vi "Motor Control Loop.vi"(8 "error in (no error)":errorcluster) -> (0 "error out":errorcluster)   [LabVIEW 2017]
uses:
  <vilib>/Simulation/Scripting/Companion Diagram/SimConfigNode/SimParams.ctl
  <vilib>/Simulation/Scripting/Companion Diagram/SimConfigNode/_simSolvers.ctl
  <vilib>/Simulation/Implementation/Shared/SIMSCR Execution Mode.ctl
  <vilib>/Platform/TimedLoop/XDataNode/timing_clust.ctl
  <vilib>/Platform/TimedLoop/XDataNode/nitl_modes.ctl
  <vilib>/Platform/TimedLoop/XDataNode/wakeup.ctl
  <vilib>/Simulation/Param Hierarchy/Typedefs/SIMPH Param Control Actions.ctl
  <vilib>/Simulation/Implementation/Shared/SIM limit type.ctl
  <vilib>/Simulation/Scripting/Editor Utilities/SIM subVI tag data.ctl
  <vilib>/Simulation/Scripting/Editor Utilities/SIM subVI execution type.ctl
  <vilib>/Simulation/Implementation/Shared/NILVSim_ParamChanged.vi
  <vilib>/Simulation/Implementation/Shared/NILVSim_FinishedLate.vi
  <vilib>/Simulation/Implementation/Shared/NILVSIM_BeginStep.vi
  <vilib>/Simulation/Utility/Implementation/SIM Halt.vi
  <vilib>/Simulation/SignalArithmetic/Implementation/NILVSim Gain.llb/SIM Gain (vector,ScalarGain).vi
  <vilib>/Simulation/ContinuousLinear/Implementation/NILVSim Integrator new.llb/SIM Integrator distributor (scalar).vi
  <vilib>/Simulation/ContinuousLinear/Implementation/NILVSim Integrator new.llb/SIM Integrator Distributor (vector).vi
  <vilib>/Simulation/Implementation/Shared/SIM Fire Discrete SubVI.vi
  <vilib>/Simulation/Nonlinear/Implementation/NILVSim Saturation.llb/SIM Saturation (scalar).vi
  <vilib>/Simulation/Nonlinear/Implementation/NILVSim Saturation.llb/SIM Saturation (vector).vi
  <vilib>/Simulation/ContinuousLinear/Implementation/NILVSim Integrator new.llb/SIM Integrator collector (scalar).vi
  <vilib>/Analysis/coordinate.llb/2D Cartesian Coordinate Rotation.vi
  <vilib>/Analysis/coordinate.llb/2D Cartesian Coordinate Rotation (Scalar).vi
  <vilib>/Simulation/ContinuousLinear/Implementation/NILVSim Integrator new.llb/SIM Integrator Collector (vector).vi
  <vilib>/Simulation/Implementation/Shared/NILVSim_Manager.vi
  <vilib>/Utility/error.llb/Clear Errors.vi
  <vilib>/Simulation/Implementation/Shared/NILVSim_FinalizeModel.vi
  <vilib>/Simulation/Implementation/Shared/SIM Fire Discrete SubVI (Core).vi
  <vilib>/robotics/Steering/Mecanum Steering Frame/NI_Robotics_Mecanum Steering Frame.lvclass
  c:/Program Files (x86)/National Instruments/LabVIEW 2017/vi.lib/robotics/Steering/Steering Frame/NI_Robotics_Steering Frame.lvclass
  <vilib>/Simulation/Implementation/Shared/SIM Unbundle Sim Info.vi
  <vilib>/Simulation/Implementation/Shared/SIMSH Read Queue.vi
  Robot Parameters/Robot Parameters.vi
  <vilib>/Simulation/Implementation/Shared/NILVSim_Initialize.vi
  <vilib>/Simulation/Utility/Implementation/NILVSim Get Time and IsAcceptedStep.vi
  Simulation/Global - Real Position.vi
  <vilib>/robotics/Steering/Steering Frame/Apply Velocity to Motors.vi
  <vilib>/robotics/Steering/Steering Frame/Apply Steering Frame Velocity to Motors.vi
  Unsaturate Commanded Motor Velocities.vi
  <vilib>/robotics/Steering/Steering Frame/Get Velocity from Motors.vi
  <vilib>/robotics/Steering/Steering Frame/Get Steering Frame Velocity from Motors.vi
  <vilib>/Simulation/Implementation/Shared/NILVSim_GetModelError.vi
  <vilib>/Simulation/Implementation/Shared/SIM Bundle Sim Info.vi
  <vilib>/Simulation/Scripting/Companion Diagram/SimConfigNode/SimDog.xnode
  PID_scalar (derivative acts only on process variable).vi
  Simulation/Mecanum Robot Body Model.vi
  Simulation/Motor Model.vi
  Simulation/PID_vector (derivative acts only on process variable).vi
  <vilib>/Platform/TimedLoop/XDataNode/XDataNode.xnode
  <vilib>/Simulation/Implementation/XNodeFramework/SimXNode/SimX.xnode
  <vilib>/robotics/Utilities/NI_Robotics Utilities.lvlib
  <vilib>/Analysis/NI_AALPro.lvlib
  <vilib>/robotics/Steering/Steering Frame/NI_Robotics_Steering Frame.lvclass
  c:/Program Files (x86)/National Instruments/LabVIEW 2017/vi.lib/robotics/Steering/Special Steering Frame/NI_Robotics_Special Steering Frame.lvclass
  <vilib>/Simulation/ContinuousLinear/Implementation/NILVSim Integrator new.llb/SIM Integrator (scalar).vi
  <vilib>/Simulation/ContinuousLinear/Implementation/NILVSim Integrator new.llb/SIM Integrator (vector).vi
  <vilib>/Platform/TimedLoop/XDataNode/XDNodeRunTimeDep.lvlib
  <vilib>/Simulation/Implementation/Shared/NI_SIM_Implementation.lvlib
panel:
  in  "stop?":bool
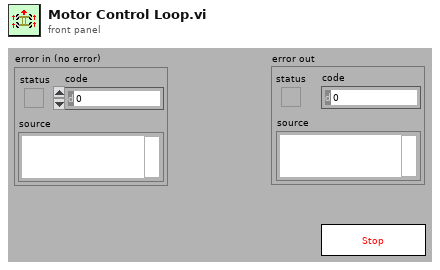
[diagram p1: front panel]
types:
  T1 = typedef "SIMSCR Execution Mode.ctl" = enum16{"Simulate to Completion", "Single Time-Step Simulation (Fixed Step Only)"}
  T2 = typedef "XDNodeRunTimeDep.lvlib/timing_clust.ctl" = cluster{"Expected End [f-1]":u64, "Actual End [f-1]":u64, "Finished Late? [f-1]":bool, "Expected End [i-1]":u64, "Actual End [i-1]":u64, "Finished Late? [i-1]":bool, "Expected Start [i]":u64, "Actual Start [i]":u64, "Expected Start [f]":u64, "Actual Start [f]":u64, "Source Name":string, "Structure Name":string, "Period":i64, "Deadline":i64, "Offset":i64, "Start":i64, "Priority":i32, "Timeout":i32, "Mode":T3, "Wakeup Reason":T4, "Error":errorcluster, "Source Type":string, "Secondary Source Type":string, "Global End Time":u64, "Global Start Time":u64, "Frame Duration":u64, "Iteration Duration":u64, "Assigned CPU":i32, "I/O Scan Engine Mode":u32}
  T3 = typedef "XDNodeRunTimeDep.lvlib/nitl_modes.ctl" = enum32{"No Change", "Process missed periods, maintain original phase", "Discard missed periods, maintain original phase", "Process missed periods, ignore original phase", "Discard missed periods, ignore original phase"}
  T4 = typedef "XDNodeRunTimeDep.lvlib/wakeup.ctl" = enum32{"Normal", "Aborted", "Asynchronous wakeup", "Timing source error", "Timed loop error", "Timeout"}
  T5 = typedef "SIMPH Param Control Actions.ctl" = enum16{"get params", "set params"}
  T6 = typedef "SIM subVI tag data.ctl" = cluster{"period":dbl, "skew":dbl, "Simulation execution type":T7}
  T7 = typedef "SIM subVI execution type.ctl" = enum16{"Function call", "Discrete", "Continuous", "Initialization only", "Final step only"}
  T8 = typedef "SIM limit type.ctl" = enum16{"upper", "lower", "both", "none"}
  T9 = cluster{"SIMSH Sim Time":dbl, "Integrator":cluster{"output":dbl}, "Gain":cluster{"output":dbl}, "Summation":cluster{"Result":dbl}, "Derivative":cluster{"output":dbl}, "Multiply":cluster{"x*y":dbl}, "Negate":cluster{"-x":dbl}, "Subtract":cluster{"x-y":dbl}, "set point":dbl, "Divide":cluster{"x/y":dbl}}
  T10 = cluster{"SIMSH Sim Time":dbl, "w":cluster{"output":dbl}, "theta":cluster{"output":dbl}, "x'":cluster{"output":dbl[]}, "x":cluster{"output":dbl[]}, "Wheel theta":cluster{"output":dbl[]}, "Robot Parameters.vi 7":cluster{"mass":dbl}, "Robot Parameters.vi 6":cluster{"inertia (Izz)":dbl}, "Robot Parameters.vi 5":cluster{"center of mass y":dbl}, "Robot Parameters.vi 4":cluster{"center of mass x":dbl}, "Robot Parameters.vi 3":cluster{"robot length":dbl}, "Robot Parameters.vi 2":cluster{"robot width":dbl}, "Robot Parameters.vi":cluster{"wheel radius":dbl}, "Divide 5":cluster{"x/y":dbl[]}, "A x B.vi 3":cluster{"A x Vector":dbl[]}, "Build Array":cluster{"appended array":dbl[]}, "Multiply 6":cluster{"x*y":dbl}, "Divide 4":cluster{"x/y":dbl}, "Add 4":cluster{"x+y":dbl}, "Index Array 4":cluster{"element":dbl}, "2D Cartesian Coordinate Rotation.vi 3":cluster{"y out":dbl, "x out":dbl}, "Multiply 5":cluster{"x*y":dbl}, "Multiply 4":cluster{"x*y":dbl}, "Add 3":cluster{"x+y":dbl}, "Add 2":cluster{"x+y":dbl}, "2D Cartesian Coordinate Rotation.vi 2":cluster{"y out":dbl, "x out":dbl}, "Replace Array Subset 2":cluster{"output array":dbl[]}, "Index Array 3":cluster{"element":dbl}, "Add":cluster{"x+y":dbl}, "Compound Arithmetic":cluster{"result":dbl}, "Multiply 3":cluster{"x*y":dbl}, "Multiply 2":cluster{"x*y":dbl}, "Multiply":cluster{"x*y":dbl}, "Index Array 2":cluster{"element":dbl}, "A x B.vi 2":cluster{"A x Vector":dbl[]}, "Divide 3":cluster{"x/y":dbl[]}, "A x B.vi":cluster{"A x Vector":dbl[]}, "Divide 2":cluster{"x/y":dbl[]}, "Replace Array Subset":cluster{"output array":dbl[]}, "Negate":cluster{"-x":dbl}, "Index Array":cluster{"element":dbl}, "2D Cartesian Coordinate Rotation.vi":cluster{"y out":dbl, "x out":dbl}, "Divide":cluster{"x/y":dbl}}
  T11 = cluster{"SIMSH Sim Time":dbl, "Gain":cluster{"output":dbl[]}, "Summation 2":cluster{"Result":dbl[]}, "Shaft Angle":cluster{"output":dbl[]}}
  T12 = cluster{"SIMSH Sim Time":dbl, "Integrator":cluster{"output":dbl[]}, "Gain":cluster{"output":dbl[]}, "Summation":cluster{"Result":dbl[]}, "Derivative":cluster{"output":dbl[]}, "Multiply":cluster{"x*y":dbl[]}, "Negate":cluster{"-x":dbl[]}, "Subtract":cluster{"x-y":dbl[]}, "set point":dbl[], "Divide":cluster{"x/y":dbl[]}}
  T13 = typedef "SimParams.ctl" = cluster{"Initial Time (s)":dbl, "Final Time (s)":dbl, "Step Size (s)":dbl, "ODE Solver":T14, "Minimum Step Size (s)":dbl, "Maximum Step Size (s)":dbl, "Relative Tolerance":dbl, "Absolute Tolerance":dbl, "Software Timing":bool, "Initial Step Size (s)":dbl, "Automatic Fixed Step Size?":bool, "Automatic Discrete Step Size?":bool, "Discrete Step Size (s)":dbl, "Calculate using Time Step":bool, "Solver Wired?":bool, "Prev.Frm.Expected End":u64, "Prev.Frm.Actual End":u64, "Prev.Frm.Finished Late?":bool, "Prev.Iter.Expected End":u64, "Prev.Iter.Actual End":u64, "Prev.Iter.Finished Late?":bool, "Expected Iteration Start":u64, "Actual Iteration Start":u64, "Expected Frame Start":u64, "Actual Frame Start":u64, "Source Name":string, "Name":string, "Period":i64, "Deadline":i64, "Offset":i64, "Start":i64, "Priority":i32, "Timeout":i32, "Processor":i32, "Mode":enum32{"No Change", "Process missed periods, maintain original phase", "Discard missed periods, maintain original phase", "Process missed periods, ignore original phase", "Discard missed periods, ignore original phase"}, "Wakeup reason":enum32{"Normal", "Aborted", "Asynchronous wakeup", "Timing source error", "Timed loop error", "Timeout"}, "Error":errorcluster, "Source Type":string, "Secondary Source Type":string, "Global End Time":u64, "Global Start Time":u64, "Full Solver Reset":bool, "Execution Mode":T1, "Nan/Inf Check":bool, "Custom Solver Library":string, "Solver Is Variable":bool, "custom solver name":string, "Signal Collection Decimation":u32}
  T14 = typedef "_simSolvers.ctl" = enum16{"Runge-Kutta 1 (Euler)", "Runge-Kutta 2", "Runge-Kutta 3", "Runge-Kutta 4", "Runge-Kutta 23 (variable)", "Runge-Kutta 45 (variable)", "BDF (variable)", "Adams-Moulton (variable)", "Rosenbrock (variable)", "Discrete States Only", "SDIRK 4 (variable)", "Radau 5 (variable)", "Radau 9 (variable)", "Radau 13 (variable)", "Radau [Variable Order] (variable)", "Gear's Method (variable)", "Linearizer", "State Query", "Trim Eval", "Custom Solver"}
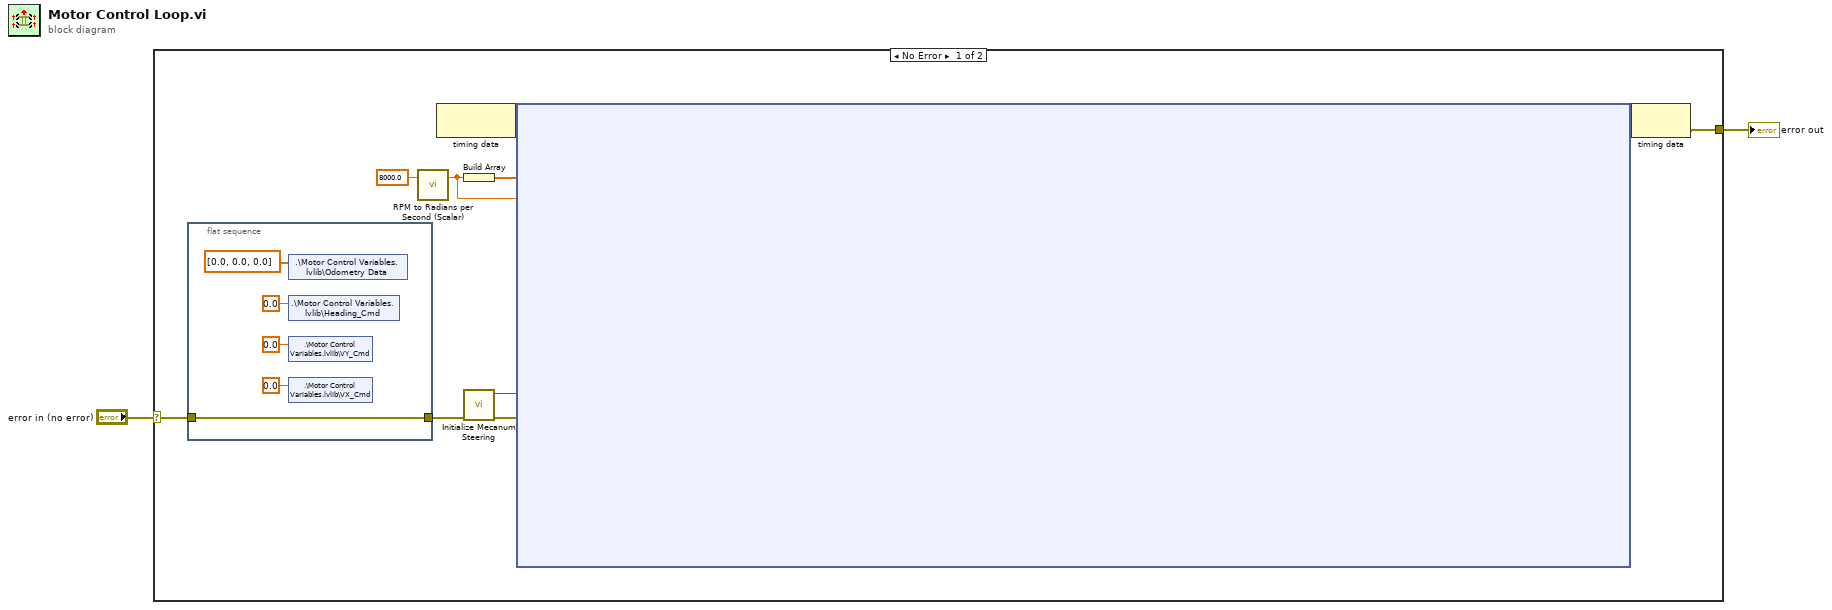
[diagram p0: block diagram]
diagram:
  n1 = case shown="No Error" "error in (no error)" {
    selector: "error in (no error)" -> [w8 w660]
    tunnel: [w6 w660] -> w1
    frame No Error {
      n2 = flat-sequence {
        tunnel: w8 -> [w13]
        tunnel: [w13] -> w4
        frame #0 {
          n3 = shared-variable ".\\Motor Control Variables.lvlib\\Odometry Data"(dbl[] [0.0, 0.0, 0.0] ("Odometry Data")) -> ()  [unwired: 1 in, 1 out]
          n4 = shared-variable ".\\Motor Control Variables.lvlib\\Heading_Cmd"(0.0 ("Heading_Cmd")) -> ()  [unwired: 1 in, 1 out]
          n5 = shared-variable ".\\Motor Control Variables.lvlib\\VY_Cmd"(0.0 ("VY_Cmd")) -> ()  [unwired: 1 in, 1 out]
          n6 = shared-variable ".\\Motor Control Variables.lvlib\\VX_Cmd"(0.0 ("VX_Cmd")) -> ()  [unwired: 1 in, 1 out]
        }
      }
      n7 = call <vilib>:"RPM to Radians per Second (Scalar).vi"("rpm"=8000.0 ("Numeric")) -> ("radians per second"=w10:dbl)  [unwired: 2 in]
      n8 = node-c288() -> (w12:variant)  [unwired: 1 in]
      n9 = Build Array(w10) -> (w9:dbl[])
      n10 = call "Initialize Mecanum Steering.vi"("error in (no error)"=w4) -> ("error out"=w5:errorcluster, "mecanum steering frame out"=w3:refnum<class "NI_Robotics_Mecanum Steering Frame.lvclass">)  [unwired: 9 in]
      n11 = node-c254 ("Simulation Loop 2")(w12, w10, w9, w5, w3) -> (w11:variant)
      n12 = node-c288(w11) -> (w6:errorcluster)
    }
    frame Error {
    }
  }
  "error out" <- w1
